vi "p2.vi"() -> ()   [LabVIEW 2025, in "d4.lvlib"]
uses:
  d4.lvlib
  <userlib>/_OpenG.lib/string/string.llb/openg_string.lvlib
  AOC/AOC.lvlib
panel:
  in  "Example":string="..@@.@@@@.\n@@@.@.@.@@\n@@@@@.@.@@\n@.@@@@..@.\n@@.@@@@.@@\n.@@@@@@@.@\n.@.@.@.@@@\n@.@@@.@@@@\n.@@@@@@@@.\n@.@.@@@.@."
  in  "Example 2":bool
  out "Answer":i64=605
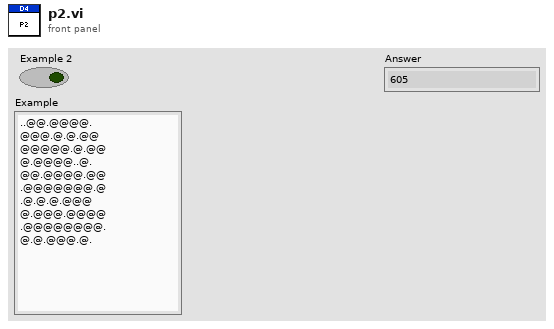
[diagram p1: front panel]
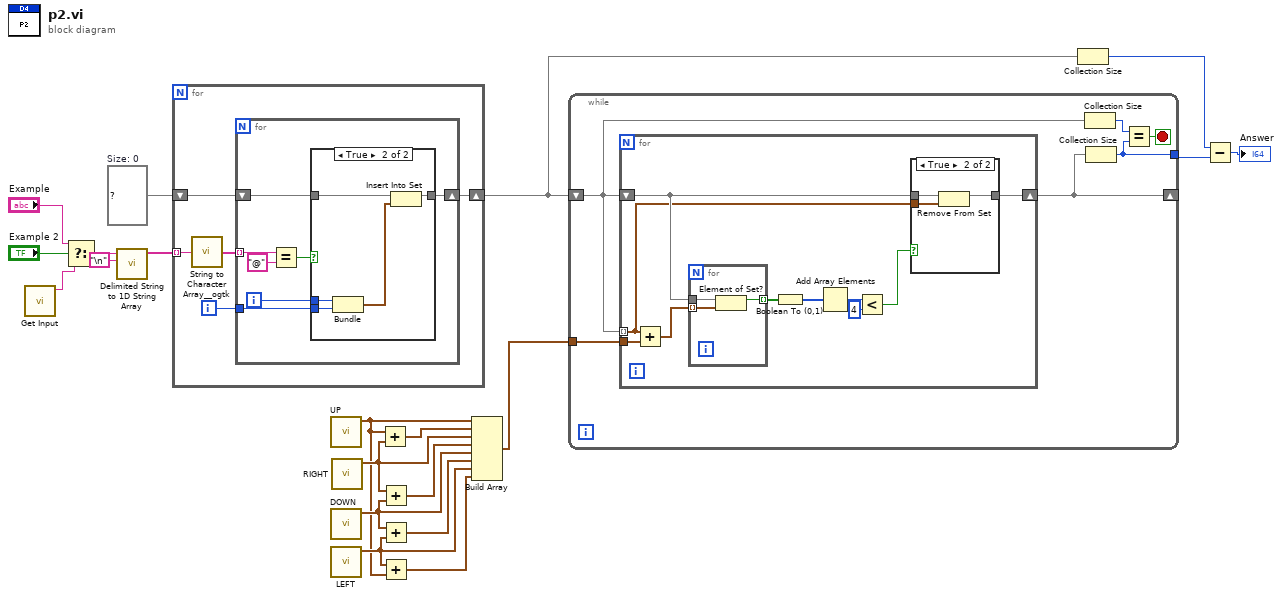
[diagram p0: block diagram]
diagram:
  w15 = set{cluster{i32, i32}} {}  # Size: 0
  n1 = call "Get Input.vi"() -> ("Input"=w20:string)  [unwired: 11 in]
  n2 = Select(t="Example", s="Example 2", f=w20) -> (s? t:f=w17:string)
  n3 = call <vilib>:"Delimited String to 1D String Array.vi"("delimiter"="\n", "delimited string"=w17) -> ("string array"=w16:string[])  [unwired: 9 in]
  n4 = for {
    tunnel: w16 -> [w25] mode=indexing
    shift-right: [w21] -> w4
    shift-left: w15 -> [w22]
    i -> [w23]
    n5 = call <userlib>:"String to Character Array__ogtk.vi"("Input String"=w25) -> ("Character Array"=w24:string[])
    n6 = for {
      tunnel: w24 -> [w32] mode=indexing
      tunnel: w23 -> [w29]
      shift-right: [w26] -> w21
      shift-left: w22 -> [w27]
      i -> [w28]
      n7 = Equal?(x=w32, y="@") -> (x = y?=w30:bool)
      n8 = case shown="True" w30 {
        tunnel: w29 -> [_ w38]
        tunnel: w28 -> [_ w37]
        tunnel: w27 -> [w33 w36]
        tunnel: [w33 w34] -> w26
        frame False {
        }
        frame True {
          n9 = Bundle(w37, w38) -> (w35:cluster{i32, i32})  [unwired: 1 in]
          n10 = Insert Into Set(10:w35, 11:w36) -> (3:w34:set{cluster{i32, i32}})  [unwired: 1 out]
        }
      }
    }
  }
  n11 = call "UP.vi"() -> ("UP"=w8:cluster{"x":i16, "y":i16})  [unwired: 11 in]
  n12 = call "DOWN.vi"() -> ("DOWN"=w10:cluster{"x":i16, "y":i16})  [unwired: 11 in]
  n13 = call "LEFT.vi"() -> ("LEFT"=w9:cluster{"x":i16, "y":i16})  [unwired: 11 in]
  n14 = call "RIGHT.vi"() -> ("RIGHT"=w13:cluster{"x":i16, "y":i16})  [unwired: 11 in]
  n15 = Add(x=w8, y=w13) -> (x+y=w14:cluster{"x":i16, "y":i16})
  n16 = Add(x=w13, y=w10) -> (x+y=w12:cluster{"x":i16, "y":i16})
  n17 = Add(x=w10, y=w9) -> (x+y=w11:cluster{"x":i16, "y":i16})
  n18 = Add(x=w9, y=w8) -> (x+y=w7:cluster{"x":i16, "y":i16})
  n19 = Build Array(w8, w14, w13, w12, w10, w11, w9, w7) -> (w6:cluster{"x":i16, "y":i16}[])
  n20 = while {
    tunnel: w6 -> [w44]
    shift-right: [w43] -> _
    shift-left: w4 -> [w42]
    tunnel: [w39] -> w3
    stop <- w40 stop-if-true
    n21 = for {
      tunnel: w42 -> [w45] mode=indexing
      tunnel: w44 -> [w54]
      shift-right: [w47] -> w43
      shift-left: w42 -> [w48]
      n22 = Add(x=w45, y=w54) -> (x+y=w53:cluster{i32, i32}[])
      n23 = for {
        tunnel: w48 -> [w61]
        tunnel: w53 -> [w60] mode=indexing
        tunnel: [w59] -> w52 mode=indexing
        n24 = Element of Set?(10:w60, 11:w61) -> (3:w59:bool)
      }
      n25 = Boolean To (0,1)(Boolean=w52) -> (0, 1=w51:i16[])
      n26 = Add Array Elements(numeric array=w51) -> (sum=w50:i16)
      n27 = Less?(x=w50, y=i16 4) -> (x < y?=w46:bool)
      n28 = case shown="True" w46 {
        tunnel: w48 -> [w55 w58]
        tunnel: [w55 w57] -> w47
        tunnel: w45 -> [_ w56]
        frame False {
        }
        frame True {
          n29 = Remove From Set(10:w56, 11:w58) -> (3:w57:set{cluster{i32, i32}})  [unwired: 1 out]
        }
      }
    }
    n30 = Collection Size(1:w42) -> (0:w41:i32)
    n31 = Collection Size(1:w43) -> (0:w39:i32)
    n32 = Equal?(x=w41, y=w39) -> (x = y?=w40:bool)
  }
  n33 = Collection Size(1:w4) -> (0:w2:i32)
  n34 = Subtract(x=w2, y=w3) -> (x-y=→"Answer":i32)
